vi "ReadFromLockin.vi"(4 "#Measurements each Frequency":i32=200, 5 "Path":path, 7 "Frequency":dbl=200.0 format="%.2f", 8 "error in 2":errorcluster, 10 "TemperatureError":dbl=200.0 format="%.2f", 11 "Temperature":dbl=200.0 format="%.2f") -> (0 "error out 2":errorcluster)   [LabVIEW 2010]
uses:
  <vilib>/Utility/file.llb/Write To Spreadsheet File (DBL).vi
  <vilib>/Analysis/NI_AALBase.lvlib
panel:
  out "Phase phi":dbl=200.0 format="%.2f"
  out "Amplitude A":dbl=200.0 format="%.2f"
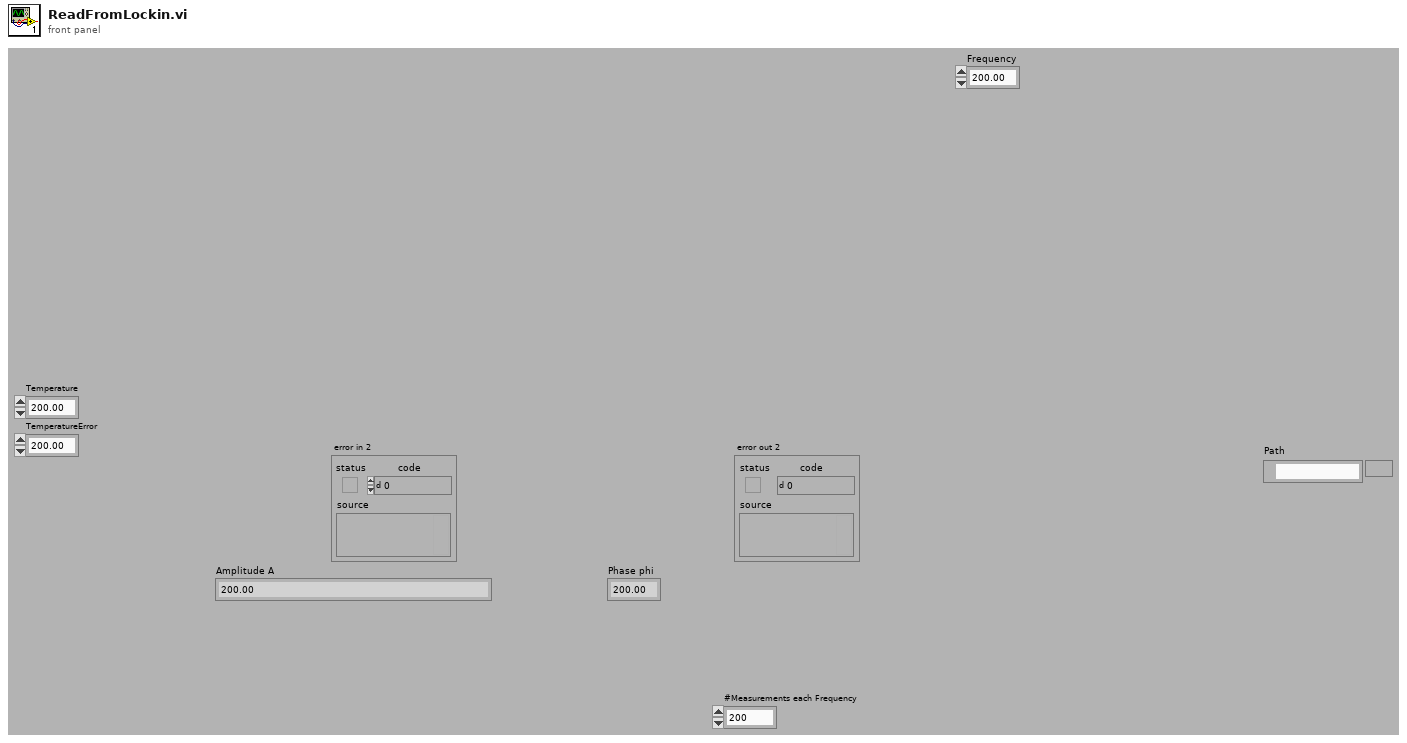
[diagram p1: front panel]
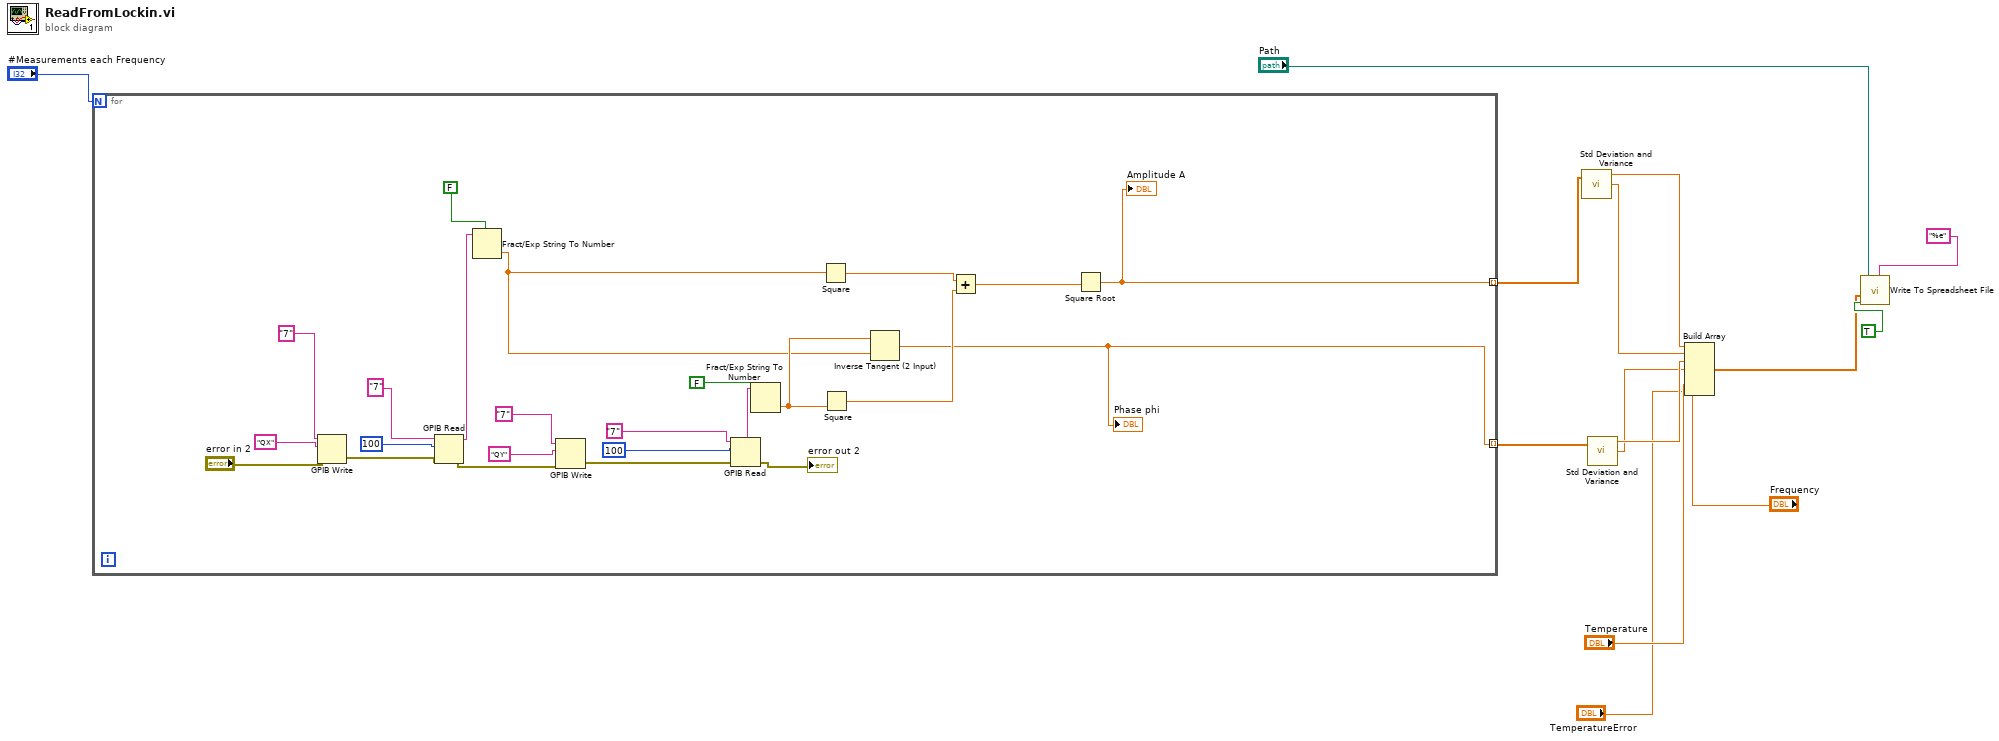
[diagram p0: block diagram]
diagram:
  n1 = for {
    N: "#Measurements each Frequency" -> [_]
    tunnel: [w16] -> w10 mode=indexing
    tunnel: [w15] -> w9 mode=indexing
    n2 = GPIB Write(0:"7", 1:"QX", 3:"error in 2") -> (6:w37:errorcluster)  [unwired: 2 in, 1 out]
    n3 = GPIB Read(0:"7", 1:100, 3:w37) -> (5:w35:string, 7:w36:errorcluster)  [unwired: 2 in, 1 out]
    n4 = Fract/Exp String To Number(use system decimal point (T)=FALSE, string=w35) -> (number=w18:dbl)  [unwired: 2 in, 1 out]
    n5 = GPIB Write(0:"7", 1:"QY", 3:w36) -> (6:w24:errorcluster)  [unwired: 2 in, 1 out]
    n6 = GPIB Read(0:"7", 1:100, 3:w24) -> (5:w21:string, 7:→"error out 2":errorcluster)  [unwired: 2 in, 1 out]
    n7 = Fract/Exp String To Number(use system decimal point (T)=FALSE, string=w21) -> (number=w32:dbl)  [unwired: 2 in, 1 out]
    n8 = Square(x=w18) -> (x^2=w17:dbl)
    n9 = Square(x=w32) -> (x^2=w31:dbl)
    n10 = Inverse Tangent (2 Input)(1:w18, 2:w32) -> (0:w15:dbl)
    "Phase phi" <- w15
    n11 = Add(x=w17, y=w31) -> (x+y=w19:dbl)
    n12 = Square Root(x=w19) -> (sqrt(x)=w16:dbl)
    "Amplitude A" <- w16
  }
  n13 = call <vilib>:"Std Deviation and Variance.vi"("X"=w10) -> ("mean"=w8:dbl, "standard deviation"=w7:dbl)  [unwired: 1 in, 1 out]
  n14 = call <vilib>:"Std Deviation and Variance.vi"("X"=w9) -> ("mean"=w5:dbl, "standard deviation"=w4:dbl)  [unwired: 1 in, 1 out]
  n15 = Build Array(w8, w7, w5, w4, "Frequency", "Temperature", "TemperatureError") -> (w6:dbl[])
  n16 = call-poly <vilib>:"Write To Spreadsheet File.vi"("format (%.3f)"="%e", "append to file? (new file:F)"=TRUE, "1D data"=w6, "file path (dialog if empty)"="Path") -> ()  [unwired: 4 in, 1 out]
